vi "读取检测值.vi"(8 "error in (no error)":errorcluster) -> (0 "error out":errorcluster, 3 "检测值":T1)   [LabVIEW 2016, in "NAQ_DO.lvlib"]
uses:
  NAQ_DO.lvlib
  <vilib>/Plasmionique/MB Master/MB_Master_Serial/MB_Master_Serial.lvclass
  C:/Program Files (x86)/National Instruments/LabVIEW 2016/vi.lib/Plasmionique/MB Master/MB_Master/MB_Master.lvclass
  <vilib>/Plasmionique/MB Master/MB Master.lvlib
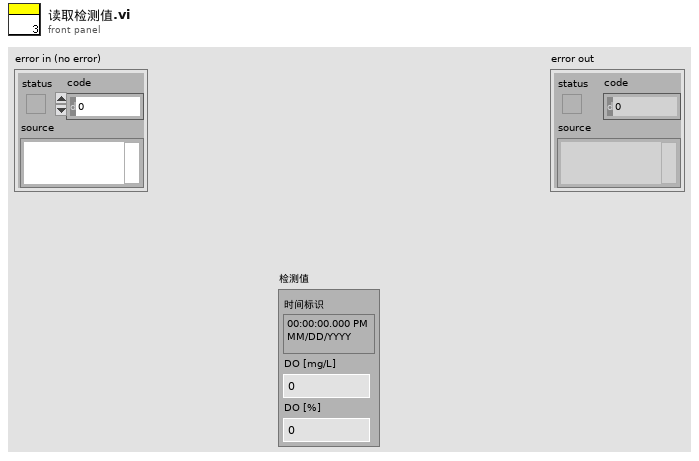
[diagram p1: front panel]
types:
  T1 = cluster{"时间标识":timestamp, "DO [mg/L]":dbl, "DO [%]":dbl}
  T2 = cluster{"seconds since 1Jan1904":timestamp, "数值":sgl, "数值":sgl}
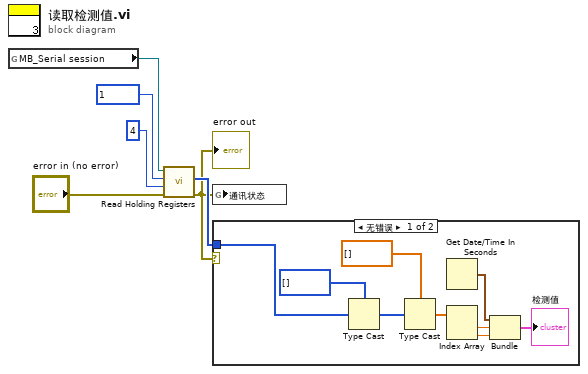
[diagram p0: block diagram]
diagram:
  n1 = global read "过程变量.vi" "MB_Serial session"() -> (w3:refnum<class "MB_Master_Serial.lvclass">)
  n2 = call <vilib>:"Read Holding Registers.vi"("error in (no error)"="error in (no error)", "quantity"=u16 4, "starting address"=u16 1, "MB session in"=w3) -> ("error out"=w1:errorcluster, "Registers"=w6:u16[])  [unwired: 5 in, 1 out]
  "error out" <- w1
  n3 = global write "过程变量.vi" "通讯状态"(w1) -> ()
  n4 = case shown="无错误" w1 {
    tunnel: w6 -> [w12 _]
    frame No Error {
      n5 = Type Cast(type=u32[] [] ("数组 2"), x=w12) -> (*(type *) &x=w13:u32[])
      n6 = Type Cast(type=sgl[] [] ("数组 2"), x=w13) -> (*(type *) &x=w11:sgl[])
      n7 = Get Date/Time In Seconds() -> (seconds since 1Jan1904=w7:timestamp)
      n8 = Index Array(array=w11) -> (element #1=w10:sgl, element #2=w9:sgl)  [unwired: 2 in]
      n9 = Bundle("seconds since 1Jan1904"=w7, "数值"=w10, "数值"=w9) -> (→"检测值":T2)  [unwired: 1 in]
    }
    frame Error {
    }
  }
